vi "公式复合写入.vi"(5 "标定时间输入":timestamp, 6 "曲线模型":T1={"标液浓度1"=0.0, "测量吸光度1"=0.0, "样品1启用"=FALSE, "标液浓度2"=0.0, "测量吸光度2"=0.0, "样品2启用"=FALSE, "标液浓度3"=0.0, "测量吸光度3"=0.0, "样品3启用"=FALSE, "标液浓度4"=0.0, "测量吸光度4"=0.0, "样品4启用"=FALSE, "标液浓度5"=0.0, "测量吸光度5"=0.0, "样品5启用"=FALSE, "模型"=enum."线性", "精度"=4.0, "XY图"=[], "拟合公式"="", "r^2"=0.0, "标样一校准时间"=timestamp(0 s since 1904-01-01), "标样二校准时间"=timestamp(0 s since 1904-01-01), "标样三校准时间"=timestamp(0 s since 1904-01-01), "标样四校准时间"=timestamp(0 s since 1904-01-01), "标样五校准时间"=timestamp(0 s since 1904-01-01), "二次方程"={"c"=0.0, "x"=0.0, "x^2"=0.0}, "标定时间"=timestamp(0 s since 1904-01-01), "拟合公式 2"="", "r^2 2"=0.0} {"r^2 2" format="%.7f"; "标定时间" format="%<%m/%d/%y %H:%M:%S>T"; "标样五校准时间" format="%<%m/%d/%y %H:%M:%S>T"; "标样四校准时间" format="%<%m/%d/%y %H:%M:%S>T"; "标样三校准时间" format="%<%m/%d/%y %H:%M:%S>T"; "标样二校准时间" format="%<%m/%d/%y %H:%M:%S>T"; "标样一校准时间" format="%<%m/%d/%y %H:%M:%S>T"; "r^2" format="%.7f"; "测量吸光度5" format="%#.6f"; "测量吸光度4" format="%#.6f"; "测量吸光度3" format="%#.6f"; "测量吸光度2" format="%#.6f"; "测量吸光度1" format="%#.6f"}, 7 "公式 2":cluster{"X^2":dbl, "X":dbl, "b":dbl}, 8 "量程下拉列表":enum16{"低量程", "高量程"}(ring), 9 "测量模式":T2(ring), 10 "临界滴定数":dbl format="%#_13g", 11 "公式":cluster{"X^2":dbl, "X":dbl, "b":dbl}) -> (3 "标定时间输出":timestamp)   [LabVIEW 2016, in "斯坦道CODMn新电路板.lvlib"]
uses:
  <vilib>/Utility/miscctls.llb/LVPointTypeDef.ctl
panel:
  in  "一键写入":bool=TRUE
  out "连接的字符串":string
  in  "参数下拉列表":enum16{"CODMn"}(ring)
  in  "取消":bool
  in  "确认":bool
  # "请选择要写入的参数"
  # "校准时间"
  # "标液浓度"
  # "吸光值显示"
  # "标液一"
  # "标液二"
  # "标液三"
  # "零点"
  # "跨度"
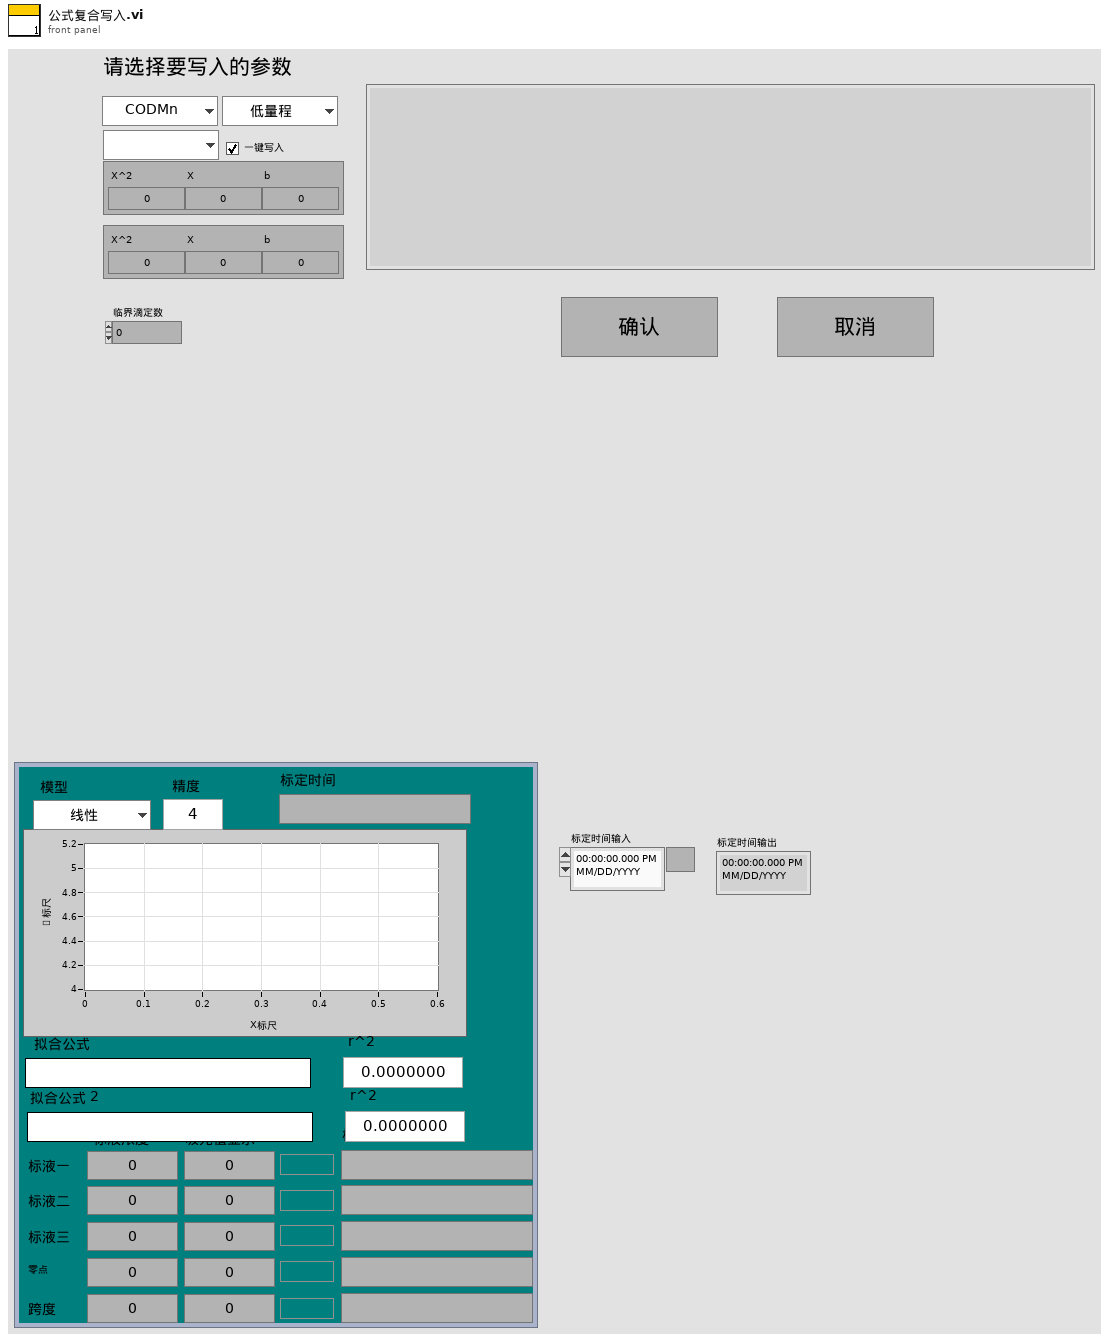
[diagram p1: front panel]
types:
  T1 = cluster{"标液浓度1":dbl, "测量吸光度1":dbl, "样品1启用":bool, "标液浓度2":dbl, "测量吸光度2":dbl, "样品2启用":bool, "标液浓度3":dbl, "测量吸光度3":dbl, "样品3启用":bool, "标液浓度4":dbl, "测量吸光度4":dbl, "样品4启用":bool, "标液浓度5":dbl, "测量吸光度5":dbl, "样品5启用":bool, "模型":enum32{"线性", "多项式", "折线"}, "精度":dbl, "XY图":cluster{"X Values":dbl[], "Y Values":dbl[]}[], "拟合公式":string, "r^2":dbl, "标样一校准时间":timestamp, "标样二校准时间":timestamp, "标样三校准时间":timestamp, "标样四校准时间":timestamp, "标样五校准时间":timestamp, "二次方程":cluster{"c":dbl, "x":dbl, "x^2":dbl}, "标定时间":timestamp, "拟合公式 2":string, "r^2 2":dbl}
  T2 = enum16{"", "水样测量", "标样核查", "零点核查", "跨度核查", "空白测试", "平行样测试", "加标回收"}
  T3 = typedef "LVPointTypeDef.ctl" = cluster{"Horizontal":i16, "Vertical":i16}
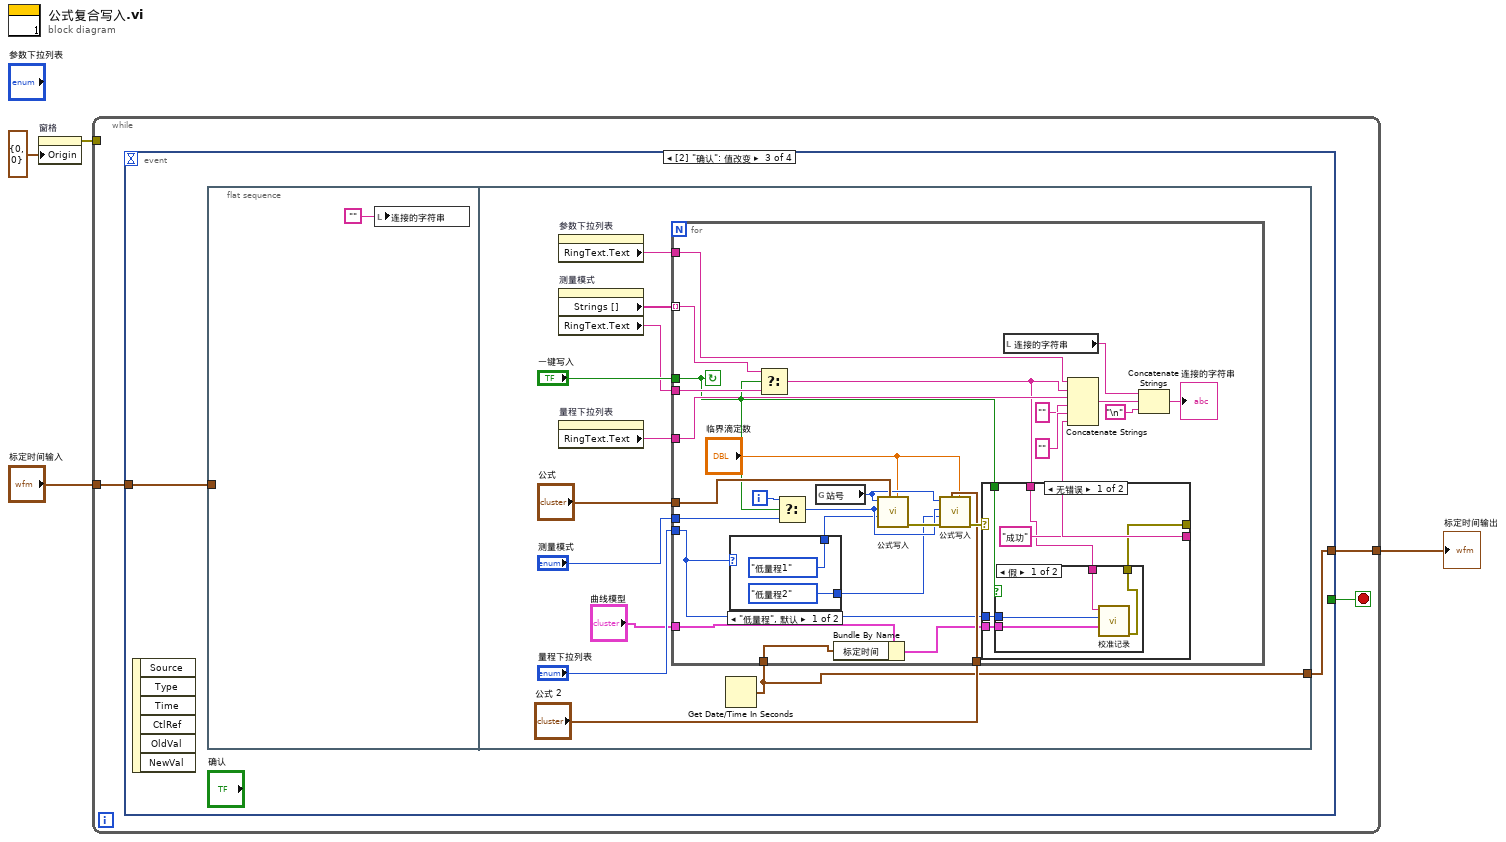
[diagram p0: block diagram]
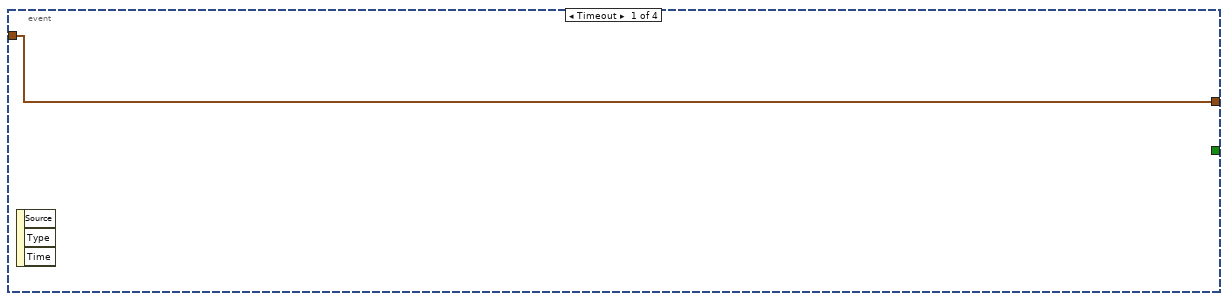
[diagram p2: hidden frame]
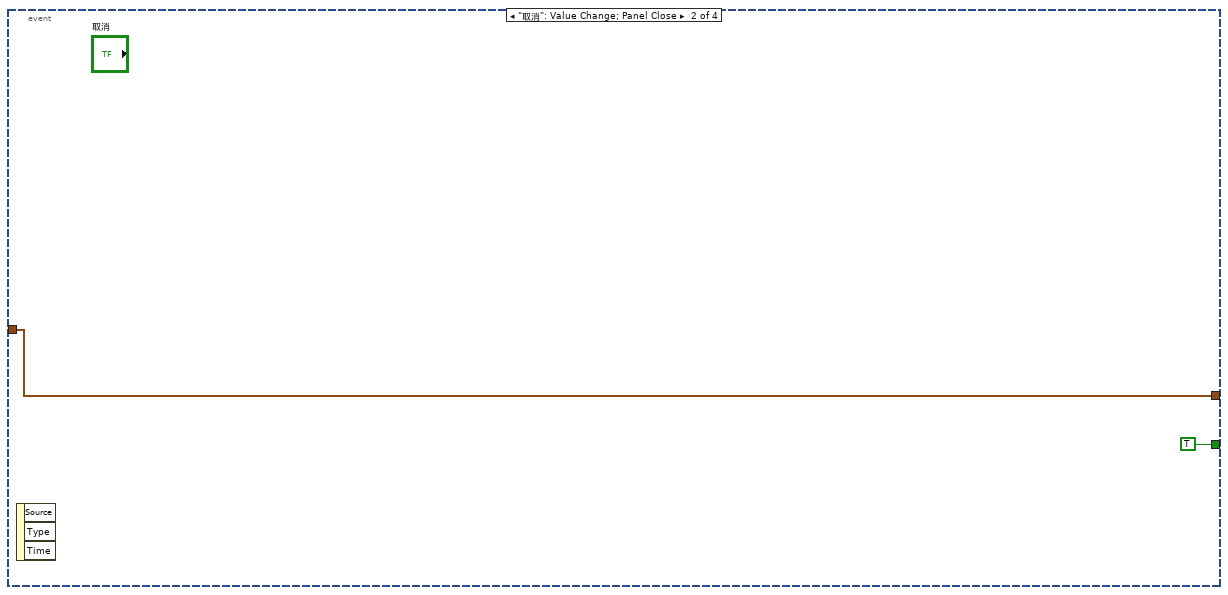
[diagram p3: hidden frame]
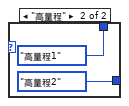
[diagram p4: hidden frame]
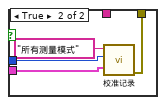
[diagram p5: hidden frame]
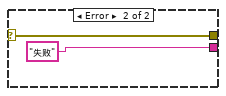
[diagram p6: hidden frame]
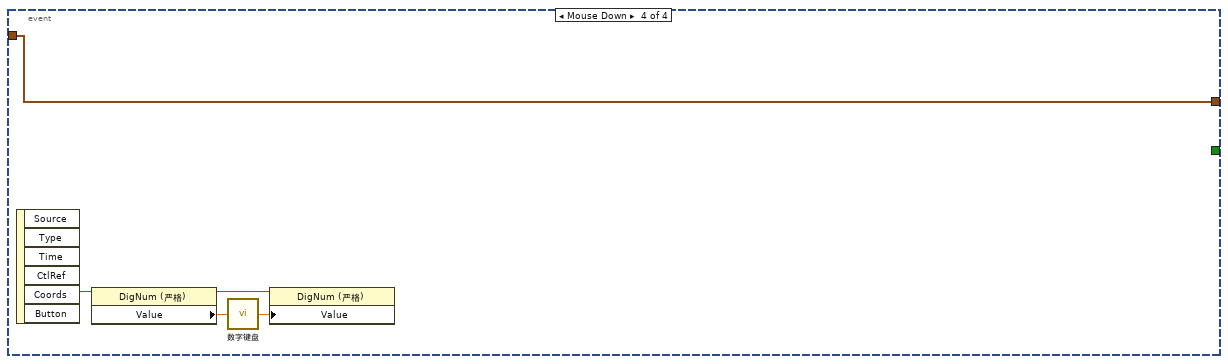
[diagram p7: hidden frame]
diagram:
  n1 = property on="窗格" class="Pane"("Origin"=T3 {"Horizontal"=0, "Vertical"=0} ("原点")) -> (error out=w3:errorcluster)  [unwired: 2 in, 1 out]
  n2 = while {
    tunnel: w3 -> [_]
    tunnel: "标定时间输入" -> [w6]
    tunnel: [w5] -> w1
    stop <- w7 stop-if-true
    n3 = event shown="[2] \"确认\": 值改变" {
      selector: _ -> [_ _ _ _]
      dyn-events: _ -> [_ _ _ _]
      timeout: _ -> [_ _ _ _]
      tunnel: [_ TRUE _ _] -> w7
      tunnel: w6 -> [w8 w9 w12 w73]
      tunnel: [w8 w9 w11 w73] -> w5
      event Timeout {
        n4 = event-data() -> ()  [unwired: 1 in, 3 out]
      }
      event "取消": Value Change; Panel Close {
        n5 = event-data() -> ()  [unwired: 1 in, 3 out]
      }
      event "确认": Value Change {
        n6 = event-data() -> ()  [unwired: 1 in, 6 out]
        n7 = flat-sequence {
          tunnel: w12 -> [_]
          tunnel: [w14] -> w11
          frame #0 {
            n8 = local write "连接的字符串"("") -> ()
          }
          frame #1 {
            n9 = property on="参数下拉列表" class="Enum (严格)"() -> ("RingText.Text"=w17:string)  [unwired: 2 in, 2 out]
            n10 = property on="测量模式" class="Enum (严格)"() -> ("Strings []"=w18:string[], "RingText.Text"=w20:string)  [unwired: 2 in, 2 out]
            n11 = property on="量程下拉列表" class="Enum (严格)"() -> ("RingText.Text"=w19:string)  [unwired: 2 in, 2 out]
            n12 = Get Date/Time In Seconds() -> (seconds since 1Jan1904=w14:timestamp)
            n13 = for {
              tunnel: "公式" -> [w38]
              tunnel: "量程下拉列表" -> [w30]
              tunnel: w18 -> [w29] mode=indexing
              tunnel: w20 -> [w50]
              tunnel: "一键写入" -> [w31]
              tunnel: "测量模式" -> [w51]
              tunnel: w17 -> [w44]
              tunnel: w19 -> [w42]
              tunnel: "公式 2" -> [w33]
              tunnel: "曲线模型" -> [w28]
              tunnel: w14 -> [w26]
              i -> [w52]
              stop <- w31 continue-if-true
              n14 = case shown="\"低量程\", 默认" w30 {
                tunnel: [enum16{"低量程1", "低量程2", "高量程1", "高量程2"}."低量程1" ("量程") enum16{"低量程1", "低量程2", "高量程1", "高量程2"}."高量程1" ("量程")] -> w35
                tunnel: [enum16{"低量程1", "低量程2", "高量程1", "高量程2"}."低量程2" ("量程") enum16{"低量程1", "低量程2", "高量程1", "高量程2"}."高量程2" ("量程")] -> w34
                frame "低量程", Default {
                }
                frame "高量程" {
                }
              }
              n15 = Select(t=w29, s=w31, f=w50) -> (s? t:f=w25:string)
              n16 = Select(t=w52, s=w31, f=w51) -> (s? t:f=w36:i32)
              n17 = global read "CODMn断电保存全局变量.vi" "站号"() -> (w37:u16)
              n18 = Bundle By Name(cluster=w28, "标定时间"=w26) -> (w27:T1)
              n19 = call "公式写入.vi"("临界滴定数"="临界滴定数", "公式"=w38, "量程"=w35, "测量模式"=w36, "测量参数"=w37) -> ("error out"=w39:errorcluster)  [unwired: 6 in]
              n20 = call "公式写入.vi"("临界滴定数"="临界滴定数", "公式"=w33, "error in (no error)"=w39, "量程"=w34, "测量模式"=w36, "测量参数"=w37) -> ("error out"=w40:errorcluster)  [unwired: 5 in]
              n21 = case shown="无错误" w40 {
                selector: w40 -> [_ w72]
                tunnel: [w58 w72] -> _
                tunnel: ["成功" "失败"] -> w45
                tunnel: w31 -> [w61 _]
                tunnel: w30 -> [w60 _]
                tunnel: w27 -> [w59 _]
                tunnel: w25 -> [w57 _]
                frame No Error {
                  n22 = case shown="假" w61 {
                    tunnel: w60 -> [w66 w70]
                    tunnel: w59 -> [w64 w69]
                    tunnel: [w63 w68] -> w58
                    tunnel: w57 -> [w65 _]
                    frame False {
                      n23 = call "校准记录.vi"("曲线模型"=w64, "量程"=w66, "测量模式"=w65) -> ("error out"=w63:errorcluster)  [unwired: 8 in]
                    }
                    frame True {
                      n24 = call "校准记录.vi"("曲线模型"=w69, "量程"=w70, "测量模式"="所有测量模式") -> ("error out"=w68:errorcluster)  [unwired: 8 in]
                    }
                  }
                }
                frame Error {
                }
              }
              n25 = local read "连接的字符串"() -> (w46:string)
              n26 = Concatenate Strings(w44, w25, w42, "" ("字符串"), "", w45) -> (w48:string)
              n27 = Concatenate Strings(w46, w48, "\n") -> (→"连接的字符串":string)
            }
          }
        }
      }
      event "公式.X^2", "公式.X", "公式.b": Mouse Down {
        n28 = event-data() -> ("CtlRef"=w77:refnum<vi>)  [unwired: 1 in, 5 out]
        n29 = property class="DigNum (严格)"(reference=w77) -> (reference out=w74:refnum<vi>, "Value"=w76:dbl)  [unwired: 1 in, 1 out]
        n30 = call "数字键盘.vi"("OldNumber"=w76) -> ("NewNumber"=w75:dbl)
        n31 = property class="DigNum (严格)"(reference=w74, "Value"=w75) -> ()  [unwired: 1 in, 2 out]
      }
    }
  }
  "标定时间输出" <- w1
